vi "PH_Cont-601k_PSU.Dev Set Charge.vi"(0 "VI in":refnum<vi>, 5 "error in (no error)":errorcluster) -> (14 "VI out":refnum<vi>, 18 "Device Error out":errorcluster, 19 "error out":errorcluster)   [LabVIEW 2014, in "PH_Cont-601k_PSU.lvlib"]
uses:
  PH_Cont-601k_PSU.lvlib
  instr.lib/pu601k/Continuum PU610K.lvlib
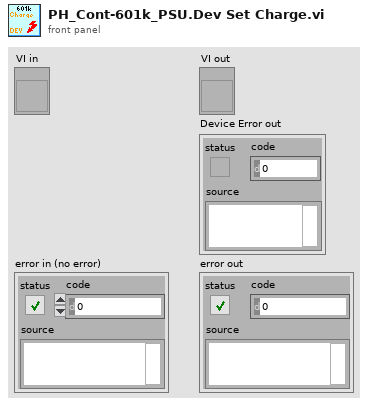
[diagram p1: front panel]
types:
  T1 = typedef "PH_Cont-601k_PSU.lvlib/PH_Cont-601k_PSU.i attribute.ctl" = cluster{"GUI Refs":T2, "Interlock":bool, "Service ID applied Voltage":i32, "Device Settings":cluster{"Configuration":T3, "Flash Interval [s]":dbl, "Mode":T4, "Voltage [V]":u16, "Charge":bool, "VISA resource name":refnum<visa-resource-name>}, "Readyness":T5, "Information":cluster{"VISA resource name":refnum<visa-resource-name>, "Tagname Power On":string, "Interlock":cluster{"Instance":string, "Tagname":string}, "Limits [V]":cluster{"Lower":dbl, "Upper":dbl}, "Tagname PSU On":string}, "R2S":bool, "Charge is allowed":bool}
  T2 = typedef "PH_Cont-601k_PSU.lvlib/PH_Cont-601k_PSU.GUI Refs.ctl" = cluster{"Power On":refnum<vi>, "Hard- and Software":refnum<vi>, "Device Status":refnum<vi>, "Device Error":refnum<vi>, "Configuration":refnum<vi>, "Flash Interval [s]":refnum<vi>, "Interlock":refnum<vi>, "Interlock Indicator":refnum<vi>, "Voltage [V]":refnum<vi>, "Readyness":refnum<vi>, "Mode":refnum<vi>, "Reset Error":refnum<vi>, "Expert working":refnum<vi>, "Charge":refnum<vi>, "PSU On":refnum<vi>}
  T3 = typedef "PH_Cont-601k_PSU.lvlib/PH_Cont-601k_PSU.Configuration.ctl" = u16
  T4 = typedef "PH_Cont-601k_PSU.lvlib/PH_Cont-601k_PSU.Mode.ctl" = enum32{"STOP", "STANDBY", "READY", "EMISSION", "ERROR"}
  T5 = typedef "PH_Cont-601k_PSU.lvlib/PH_Cont-601k_PSU.Readyness.ctl" = cluster{"Program":T6, "Device":T7}
  T6 = typedef "PH_Cont-601k_PSU.lvlib/PH_Cont-601k_PSU.Readyness Program.ctl" = enum32{"OFF", "POWER", "INTERLOCK"}
  T7 = typedef "PH_Cont-601k_PSU.lvlib/PH_Cont-601k_PSU.Readyness Device.ctl" = enum32{"OFF", "CONNECTING", "CONNECTED", "OPERATING", "EOC", "ERROR"}
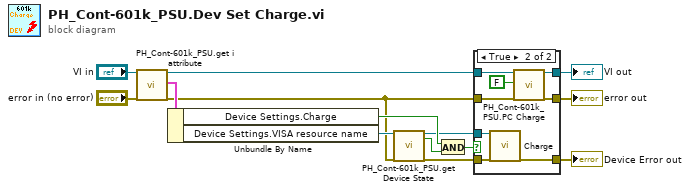
[diagram p0: block diagram]
diagram:
  n1 = call "PH_Cont-601k_PSU.get i attribute.vi"("i ref in"="VI in", "error in (no error)"="error in (no error)") -> ("i ref out"=w11:refnum<vi>, "i attribute"=w6:T1, "error out"=w1:errorcluster)  [unwired: 15 in]
  n2 = Unbundle By Name(w6) -> ("Device Settings.Charge"=w10:bool, "Device Settings.VISA resource name"=w9:refnum<visa-resource-name>)
  n3 = call "PH_Cont-601k_PSU.get Device State.vi"("VISA Refnum in"=w9, "Device Error in"=w1) -> ("VISA Refnum out"=w7:refnum<visa-resource-name>, "Charge is allowed"=w2:bool, "Device Error out"=w8:errorcluster)  [unwired: 9 in, 6 out]
  n4 = And(x=w10, y=w2) -> (x .and. y?=w5:bool)
  n5 = case shown="True" w5 {
    tunnel: w8 -> [w17 w25]
    tunnel: w7 -> [_ w24]
    tunnel: [w17 w23] -> w12
    tunnel: w1 -> [w15 w22]
    tunnel: w11 -> [w16 w21]
    tunnel: [w16 w20] -> w13
    tunnel: [w15 w19] -> w14
    frame False {
    }
    frame True {
      n6 = call "Charge.vi"("VISA resource name"=w24, "error in"=w25) -> ("error out"=w23:errorcluster)  [unwired: 16 in, 1 out]
      n7 = call "PH_Cont-601k_PSU.PC Charge.vi"("VI in"=w21, "Charge"=FALSE, "error in (no error)"=w22) -> ("VI out"=w20:refnum<vi>, "error out"=w19:errorcluster)  [unwired: 14 in, 1 out]
    }
  }
  "error out" <- w14
  "VI out" <- w13
  "Device Error out" <- w12
